vi "Destroy Request Events.vi"(8 "error in":errorcluster) -> (0 "error out":errorcluster)   [LabVIEW 2022 SP3, in "MainPanel.lvlib"]
doc: "Destroy the requests user events, even if there is an incoming error.\n\n<b>NOTE</b>: The contents of this VI are automatically generated and modified by the <b>Tools > DQMH Consortium > DQMH</b> utilities. Consider using those utilities instead of making your own modifications to this VI.\n_____\nBased on DQMH Project Template 7.0.1.1316."
uses:
  MainPanel.lvlib
panel:
  # "NOTE: The contents of this VI are automatically generated and modified by the Tools > DQMH Consortium > DQMH utilities. Consider using those utilities instead of making your own modifications to this VI."
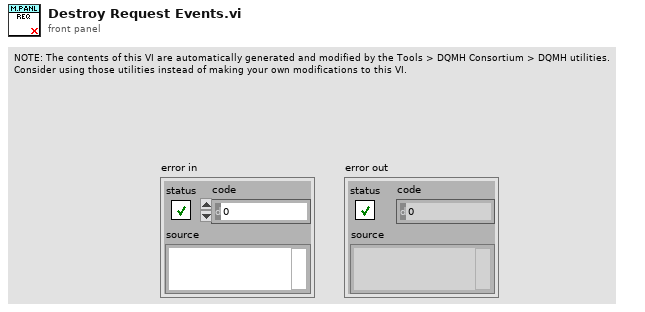
[diagram p1: front panel]
types:
  T1 = typedef "MainPanel.lvlib/Request Events--cluster.ctl" = cluster{"Stop Module":refnum<user-event>, "Do Something":refnum<user-event>, "Do Something Else":refnum<user-event>, "Do Something Else and Wait for Reply":refnum<user-event>, "Show Panel":refnum<user-event>, "Hide Panel":refnum<user-event>, "Get Module Execution Status":refnum<user-event>, "Show Diagram":refnum<user-event>, "Prepare":refnum<user-event>, "Configure":refnum<user-event>, "Request UI Display":refnum<user-event>, "Private":cluster{"Update UI":refnum<user-event>}}
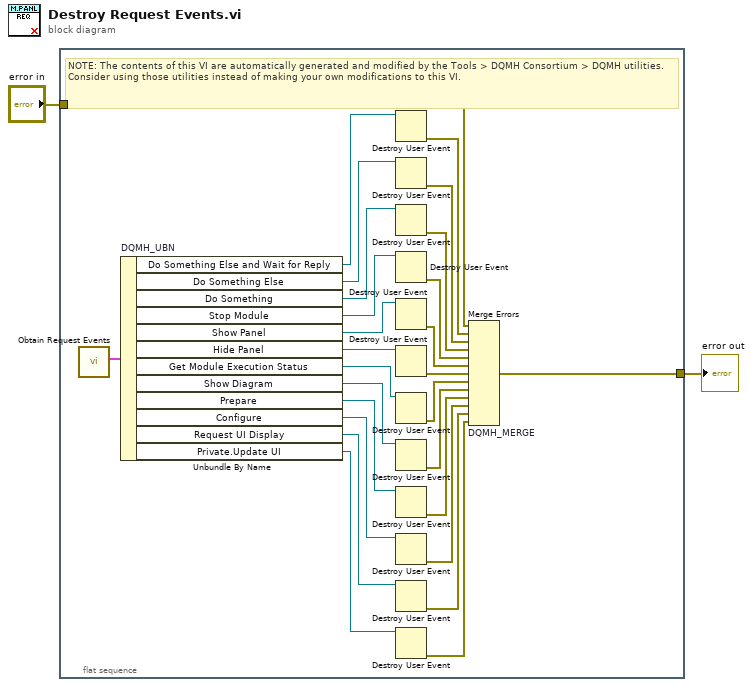
[diagram p0: block diagram]
diagram:
  n1 = flat-sequence {
    tunnel: [w28] -> w2
    tunnel: "error in" -> [w15]
    frame #0 {
      # "NOTE: The contents of this VI are automatically generated and modified by the Tools > DQMH Consortium > DQMH utilities. Consider using those utilities instead of making your own modifications to this VI."
      n2 = call "Obtain Request Events.vi"() -> ("MainPanel Request Events"=w27:T1)  [unwired: 10 in, 1 out]
      n3 = Unbundle By Name "DQMH_UBN"(w27) -> ("Do Something Else and Wait for Reply"=w17:refnum<user-event>, "Do Something Else"=w23:refnum<user-event>, "Do Something"=w25:refnum<user-event>, "Stop Module"=w26:refnum<user-event>, "Show Panel"=w19:refnum<user-event>, "Hide Panel"=w18:refnum<user-event>, "Get Module Execution Status"=w13:refnum<user-event>, "Show Diagram"=w11:refnum<user-event>, "Prepare"=w9:refnum<user-event>, "Configure"=w7:refnum<user-event>, "Request UI Display"=w5:refnum<user-event>, "Private.Update UI"=w3:refnum<user-event>)
      n4 = Destroy User Event(user event=w17) -> (error out=w16:errorcluster)  [unwired: 1 in]
      n5 = Destroy User Event(user event=w23) -> (error out=w22:errorcluster)  [unwired: 1 in]
      n6 = Destroy User Event(user event=w25) -> (error out=w24:errorcluster)  [unwired: 1 in]
      n7 = Destroy User Event(user event=w26) -> (error out=w29:errorcluster)  [unwired: 1 in]
      n8 = Destroy User Event(user event=w19) -> (error out=w21:errorcluster)  [unwired: 1 in]
      n9 = Destroy User Event(user event=w18) -> (error out=w20:errorcluster)  [unwired: 1 in]
      n10 = Destroy User Event(user event=w13) -> (error out=w14:errorcluster)  [unwired: 1 in]
      n11 = Destroy User Event(user event=w11) -> (error out=w12:errorcluster)  [unwired: 1 in]
      n12 = Destroy User Event(user event=w9) -> (error out=w10:errorcluster)  [unwired: 1 in]
      n13 = Destroy User Event(user event=w7) -> (error out=w8:errorcluster)  [unwired: 1 in]
      n14 = Destroy User Event(user event=w5) -> (error out=w6:errorcluster)  [unwired: 1 in]
      n15 = Destroy User Event(user event=w3) -> (error out=w4:errorcluster)  [unwired: 1 in]
      n16 = Merge Errors "DQMH_MERGE"(w15, w16, w22, w24, w29, w21, w20, w14, w12, w10, w8, w6, w4) -> (w28:errorcluster)
    }
  }
  "error out" <- w2
